vi "Teardown.vi"() -> (2 "Msg Strategy":refnum<class "Msg Strategy.lvclass">)   [LabVIEW 2021, in "jettl.lvlib" / "Teardown Msg Strategy.lvlib"]
uses:
  Teardown Msg Strategy.lvlib
  Teardown Msg Strategy/Teardown Msg Strategy.lvclass
  C:/git/jettl/jettl/Teardown Msg Strategy/Teardown Msg Strategy/Teardown Msg Strategy.lvclass
  C:/git/jettl/jettl/jettl/Msg Strategy/Msg Strategy.lvclass
  Msg Strategy/Msg Strategy.lvclass
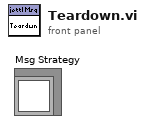
[diagram p1: front panel]
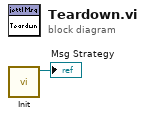
[diagram p0: block diagram]
diagram:
  n1 = call "Init.vi"() -> ("Teardown Msg Strategy out"=→"Msg Strategy":refnum<class "Teardown Msg Strategy.lvclass">)  [unwired: 11 in]
